vi "DOE Open Network Location.vi"(8 "error in (no error)":errorcluster, 11 "LV Program":T1=enum."DOE Stand") -> (0 "error out":errorcluster, 3 "Check Folder Output":enum16{"", "No", "Yes"}(ring))   [LabVIEW 2016, in "File Setup.lvlib"]
doc: "This VI prompts the user to open the network location. Generally, its not a problem, but with out a network connection, it allows the program to still run"
uses:
  File Setup.lvlib
  Custom Pallet Controls/Custom Pallet Forward.ctl
  Type Definition/Save File DOE LabView Program.ctl
panel:
  in  "OK":T2
  in  "Check Folder?":enum16{"", "No", "Yes"}(ring)
  out "Description":string="Check Network Folder?"
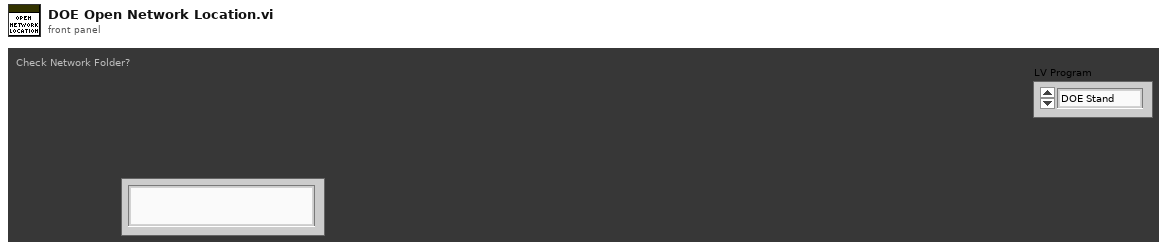
[diagram p1: front panel]
types:
  T1 = typedef "File Setup.lvlib/Save File DOE LabView Program.ctl" = enum16{"No Name Found", "DOE Stand", "Dishwasher Kitchen", "Portable Stand", "HEWH", "Dryer", "Dryer WILT", "HCC", "PRAT", "HEWH RLT"}
  T2 = typedef "Custom Pallet Forward.ctl" = bool
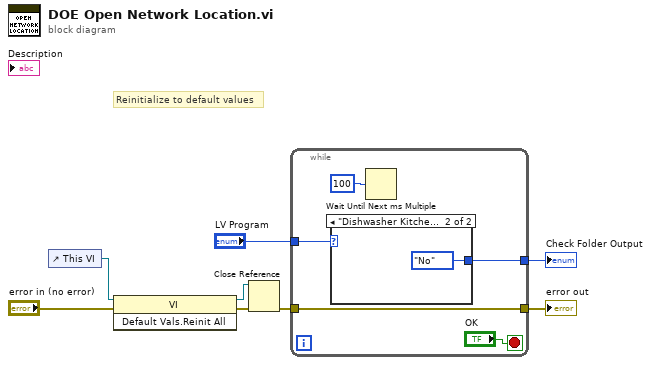
[diagram p0: block diagram]
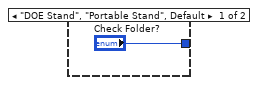
[diagram p2: hidden frame]
diagram:
  # "Reinitialize to default values"
  n1 = control-ref of="This VI"() -> (w6:refnum<vi>)
  n2 = invoke class="VI" method="Default Vals.Reinit All"(reference=w6, error in="error in (no error)") -> (reference out=w2:refnum<vi>, error out=w5:errorcluster)  [unwired: 1 in, 1 out]
  n3 = Close Reference(reference=w2, error in (no error)=w5) -> (error out=w3:errorcluster)
  n4 = while {
    tunnel: w3 -> [w11]
    tunnel: [w11] -> w8
    tunnel: [w10] -> w7
    tunnel: "LV Program" -> [w9]
    stop <- "OK" stop-if-true
    n5 = case shown="\"Dishwasher Kitchen\"" w9 {
      tunnel: ["Check Folder?" enum16{"", "No", "Yes"}."No" ("Check Folder?")] -> w10
      frame "DOE Stand", "Portable Stand", Default {
      }
      frame "Dishwasher Kitchen" {
      }
    }
    n6 = Wait Until Next ms Multiple(millisecond multiple=u32 100) -> ()  [unwired: 1 out]
  }
  "error out" <- w8
  "Check Folder Output" <- w7
